vi "FreqC.Set Gate.vi"(8 "error In":errorcluster, 10 "Gate, sec":dbl, 11 "FreqC Session in":T1) -> (0 "error out":errorcluster, 3 "FreqC Session out":T1)   [LabVIEW 2018]
uses:
  typedefs/FreqC.Session.ctl
  <instrlib>/Agilent 532XX Series/Public/Configure/Measurement/Configure Measurement (Totalize Timed).vi
  <instrlib>/Agilent 532XX Series/Agilent 532XX Series.lvlib
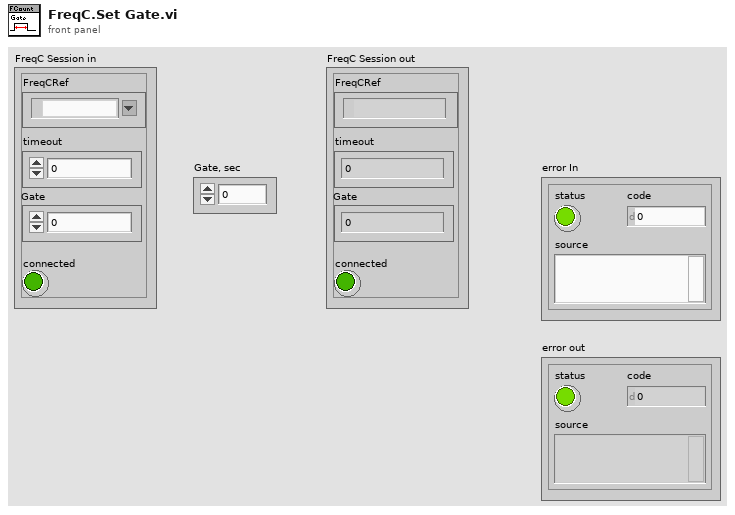
[diagram p1: front panel]
types:
  T1 = typedef "FreqC.Session.ctl" = cluster{"FreqCRef":refnum<visa-resource-name>, "timeout":dbl, "Gate":dbl, "connected":bool}
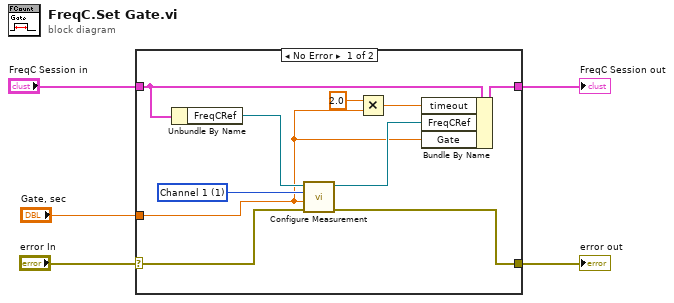
[diagram p0: block diagram]
diagram:
  n1 = case shown="No Error" "error In" {
    selector: "error In" -> [w13 w17]
    tunnel: [w12 w17] -> w4
    tunnel: "FreqC Session in" -> [w11 w16]
    tunnel: "Gate, sec" -> [w6 _]
    tunnel: [w10 w16] -> w1
    frame No Error {
      w14 = 1 items=["Channel 1"=1, "Channel 2"=2] ("Channel (1: Channel 1)")
      n2 = Unbundle By Name(w11) -> ("FreqCRef"=w15:refnum<visa-resource-name>)
      n3 = call-poly <instrlib>:"Configure Measurement.vi"("error in (no error)"=w13, "Timed Totalize (0.1 s)"=w6, "Channel (1: Channel 1)"=w14, "VISA resource name"=w15) -> ("error out"=w12:errorcluster, "VISA resource name out"=w7:refnum<visa-resource-name>)  [unwired: 6 in]
      n4 = Multiply(x=2.0, y=w6) -> (x*y=w8:dbl)
      n5 = Bundle By Name(cluster=w11, "timeout"=w8, "FreqCRef"=w7, "Gate"=w6) -> (w10:T1)
    }
    frame Error {
    }
  }
  "error out" <- w4
  "FreqC Session out" <- w1
